vi "Simple UI measurement.vi"(5 "Delay between V(in) and I(out) (ms)":u32, 7 "True voltage":bool, 8 "error in":errorcluster, 10 "Voltage in, V":dbl, 11 "VISA resource in":refnum<visa-resource-name>) -> (0 "error out":errorcluster, 1 "Current, A":dbl, 2 "Voltage out, V":dbl, 3 "VISA resource out":refnum<visa-resource-name>)   [LabVIEW 2012]
uses:
  <instrlib>/Tektronix PWS4XXX Series/Tektronix PWS4XXX Series.lvlib
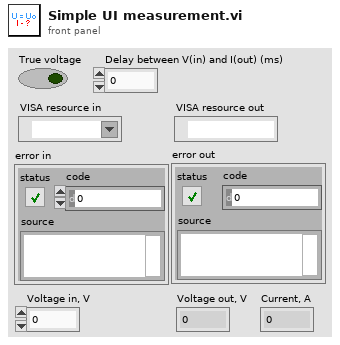
[diagram p1: front panel]
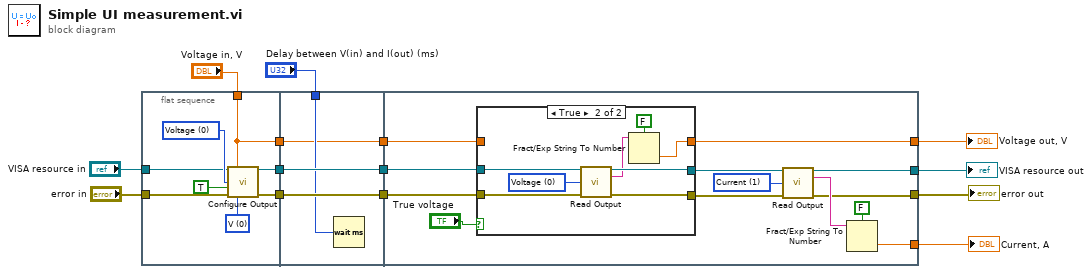
[diagram p0: block diagram]
diagram:
  n1 = flat-sequence {
    tunnel: [w20] -> w14
    tunnel: [w19] -> w13
    tunnel: "Voltage in, V" -> [w15]
    tunnel: "VISA resource in" -> [w17]
    tunnel: "error in" -> [w16]
    tunnel: [w15] -> w6
    tunnel: w14 -> [w26]
    tunnel: w13 -> [w25]
    tunnel: [w26] -> w12
    tunnel: [w25] -> w11
    tunnel: "Delay between V(in) and I(out) (ms)" -> [w24]
    tunnel: [w23] -> w7
    tunnel: w6 -> [w23]
    tunnel: w12 -> [w37]
    tunnel: w11 -> [w36]
    tunnel: w7 -> [w38]
    tunnel: [w30] -> w3
    tunnel: [w29] -> w2
    tunnel: [w28] -> w4
    tunnel: [w27] -> w5
    frame #0 {
      w21 = u16 0 items=["V", "mV", "kV", "A", "mA"] ("Unit(V)")
      w22 = u16 0 items=["Voltage", "Current"] ("Function(0:Voltage)")
      n2 = call <instrlib>:"Configure Output.vi"("VISA resource name"=w17, "Manual Range(0.00)"=w15, "Function(0:Voltage)"=w22, "Enable Output (T: Enable)"=TRUE, "error in (no error)"=w16, "Unit(V)"=w21) -> ("VISA resource name out"=w20:refnum<visa-resource-name>, "error out"=w19:errorcluster)  [unwired: 8 in]
    }
    frame #1 {
      n3 = Wait (ms)(milliseconds to wait=w24) -> ()  [unwired: 1 out]
    }
    frame #2 {
      w33 = u16 1 items=["Voltage", "Current", "Power"] ("Measurement Function (0:Voltage)")
      n4 = case shown="True" "True voltage" {
        tunnel: w38 -> [w42 _]
        tunnel: [w42 w44] -> w27
        tunnel: w37 -> [w41 w50]
        tunnel: w36 -> [w40 w49]
        tunnel: [w41 w47] -> w32
        tunnel: [w40 w46] -> w31
        frame False {
        }
        frame True {
          w48 = u16 0 items=["Voltage", "Current", "Power"] ("Measurement Function (0:Voltage)")
          n5 = call <instrlib>:"Read Output.vi"("VISA resource name"=w50, "Measurement Function (0:Voltage)"=w48, "error in (no error)"=w49) -> ("VISA resource name out"=w47:refnum<visa-resource-name>, "Measurement"=w45:string, "error out"=w46:errorcluster)  [unwired: 10 in]
          n6 = Fract/Exp String To Number(use system decimal point (T)=FALSE, string=w45) -> (number=w44:dbl)  [unwired: 2 in, 1 out]
        }
      }
      n7 = call <instrlib>:"Read Output.vi"("VISA resource name"=w32, "Measurement Function (0:Voltage)"=w33, "error in (no error)"=w31) -> ("VISA resource name out"=w30:refnum<visa-resource-name>, "Measurement"=w34:string, "error out"=w29:errorcluster)  [unwired: 10 in]
      n8 = Fract/Exp String To Number(use system decimal point (T)=FALSE, string=w34) -> (number=w28:dbl)  [unwired: 2 in, 1 out]
    }
  }
  "Voltage out, V" <- w5
  "Current, A" <- w4
  "VISA resource out" <- w3
  "error out" <- w2
